vi "Lecroy_read.vi"(2 "Inst_parameters":T1={"Kind"=enum."LeCroy", "Strings"=["LeCroy", "192.168.137.1", "C1;C2", "V;V", "0;1", "1.0;1.0"], "uint64s"=[2, 12, 1, 0, 1, 4, 3], "Doubles"=[], "DAQmx take out list"=[]}) -> (0 "Array":dbl[][](array[numeric]))   [LabVIEW 2013]
panel:
  in  "Bool2":bool
  in  "Bool1":bool
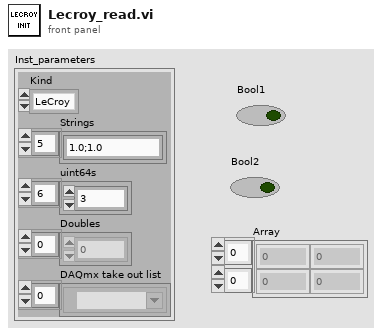
[diagram p1: front panel]
types:
  T1 = cluster{"Kind":enum16{"ADC", "K2000", "34401A", "LeCroy"}, "Strings":string[], "uint64s":u64[], "Doubles":dbl[], "DAQmx take out list":refnum<k21>[]}
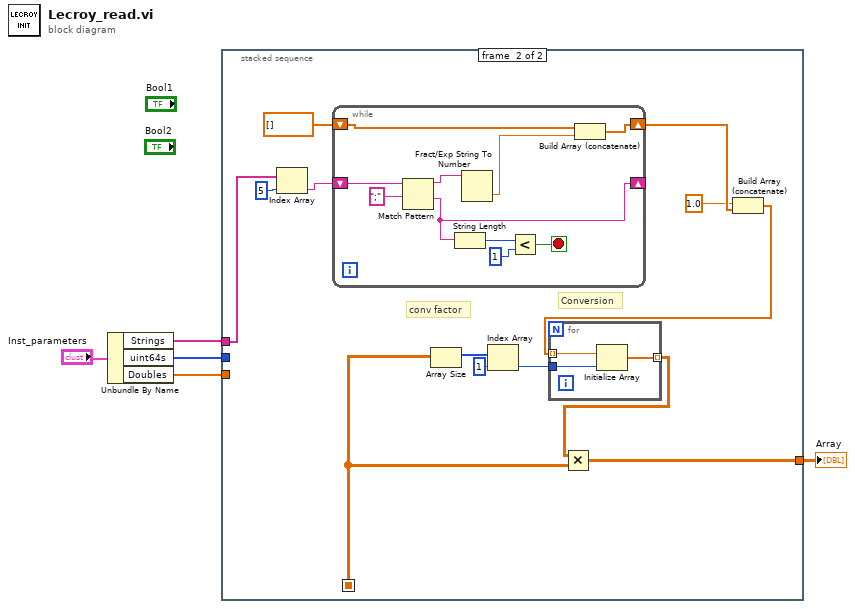
[diagram p0: block diagram]
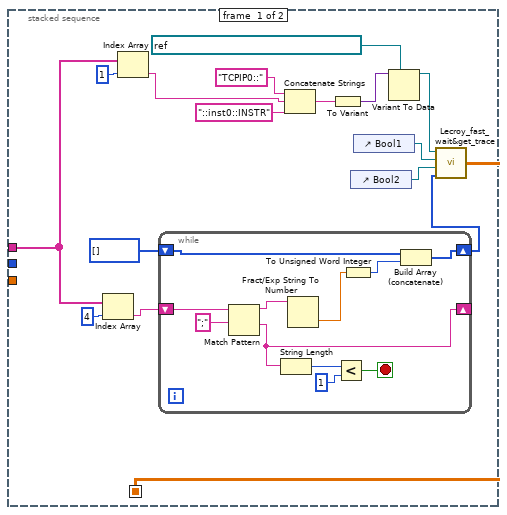
[diagram p2: hidden frame]
diagram:
  n1 = Unbundle By Name("Inst_parameters") -> ("Strings"=w4:string[], "uint64s"=w3:u64[], "Doubles"=w2:dbl[])
  n2 = stacked-sequence {
    seq-local: [w6 _] -> [_ w35]
    tunnel: w4 -> [w11 w42]
    tunnel: w3 -> [_ _]
    tunnel: w2 -> [_ _]
    tunnel: [_ w33] -> w1
    frame #0 {
      n3 = Index Array(array=w11, index=4) -> (element=w9:string)
      n4 = Index Array(array=w11, index=1) -> (element=w14:string)
      n5 = while {
        shift-right: [w24] -> w8
        shift-left: u16[] [] -> [w25]
        shift-right: [w26] -> _
        shift-left: w9 -> [w32]
        stop <- w27 stop-if-true
        n6 = Match Pattern(string=w32, regular expression=";") -> (before substring=w30:string, after substring=w26:string)  [unwired: 1 in, 2 out]
        n7 = String Length(string=w26) -> (length=w29:i32)
        n8 = Fract/Exp String To Number(string=w30) -> (number=w22:dbl)  [unwired: 3 in, 1 out]
        n9 = Less?(x=w29, y=1) -> (x < y?=w27:bool)
        n10 = To Unsigned Word Integer(number=w22) -> (unsigned 16bit integer=w23:u16)
        n11 = Build Array (concatenate)(w25, w23) -> (w24:u16[])
      }
      n12 = Concatenate Strings("TCPIP0::" ("string"), w14, "::inst0::INSTR" ("string")) -> (w19:string)
      n13 = To Variant(anything=w19) -> (Variant=w16:variant)
      n14 = control-ref of="Bool2"() -> (w13:refnum<vi>)
      n15 = control-ref of="Bool1"() -> (w21:refnum<vi>)
      n16 = Variant To Data(type=refnum<visa-resource-name> "TCPIP0::192.168.137.3::inst0::INSTR" ("VISA resource name"), Variant=w16) -> (data=w7:refnum<visa-resource-name>)  [unwired: 1 in, 1 out]
      n17 = call "Lecroy_fast_wait&get_trace.vi"("Activated channels"=w8, "stop (ref)"=w13, "start (ref)"=w21, "VISA resource name"=w7) -> ("measures"=w6:dbl[][])
    }
    frame #1 {
      # "Conversion"
      # "conv factor"
      n18 = Index Array(array=w42, index=5) -> (element=w43:string)
      n19 = while {
        shift-right: [w50] -> w38
        shift-left: dbl[] [] -> [w51]
        shift-right: [w52] -> _
        shift-left: w43 -> [w58]
        stop <- w53 stop-if-true
        n20 = Match Pattern(string=w58, regular expression=";") -> (before substring=w56:string, after substring=w52:string)  [unwired: 1 in, 2 out]
        n21 = String Length(string=w52) -> (length=w55:i32)
        n22 = Fract/Exp String To Number(string=w56) -> (number=w49:dbl)  [unwired: 3 in, 1 out]
        n23 = Less?(x=w55, y=1) -> (x < y?=w53:bool)
        n24 = Build Array (concatenate)(w51, w49) -> (w50:dbl[])
      }
      n25 = Array Size(array=w35) -> (size(s)=w41:i32[])
      n26 = Index Array(array=w41, index=1) -> (element=w39:i32)
      n27 = Build Array (concatenate)(1.0 ("number"), w38) -> (w37:dbl[])
      n28 = for {
        tunnel: w37 -> [w48] mode=indexing
        tunnel: w39 -> [w47]
        tunnel: [w46] -> w34 mode=indexing
        n29 = Initialize Array(w48, w47) -> (w46:dbl[])
      }
      n30 = Multiply(x=w34, y=w35) -> (x*y=w33:dbl[][])
    }
  }
  "Array" <- w1
